vi "Log Setpoints.vi"(8 "error in (no error)":errorcluster, 9 "Time Stamp":timestamp, 10 "Setpoints":T1, 11 "Logger in":refnum<class "Logger.lvclass">) -> (0 "error out":errorcluster, 3 "Logger out":refnum<class "Logger.lvclass">)   [LabVIEW 2015, in "Logger Actor.lvlib" / "Logger.lvclass"]
uses:
  Logger.lvclass
  <vilib>/NI/Tools/Keyed Array/KeyedArray.ctl
  Logger.lvclass/Logger.ctl
  Utilities/Message Strings.llb/Message String Utilities.lvlib
  <vilib>/NI/Tools/Keyed Array/Tools_KeyedArray.lvlib
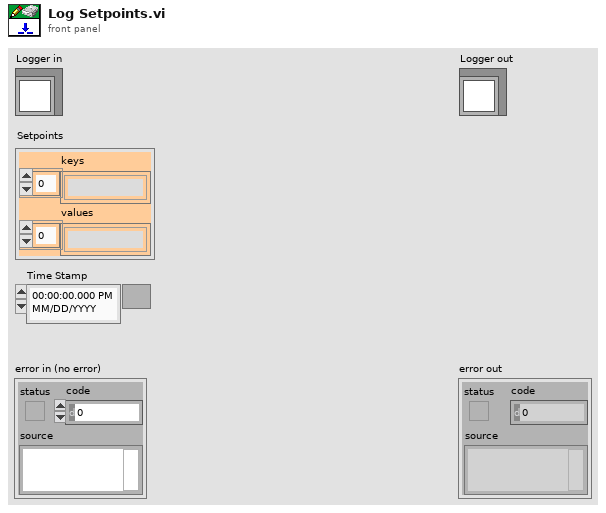
[diagram p1: front panel]
types:
  T1 = typedef "Tools_KeyedArray.lvlib/KeyedArray.ctl" = cluster{"keys":string[], "values":string[]}
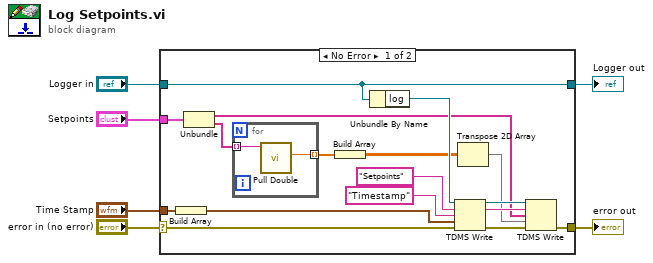
[diagram p0: block diagram]
diagram:
  n1 = case shown="No Error" "error in (no error)" {
    selector: "error in (no error)" -> [w8 w27]
    tunnel: [w12 w27] -> w5
    tunnel: [w23 w26] -> w3
    tunnel: "Logger in" -> [w23 w26]
    tunnel: "Time Stamp" -> [w19 _]
    tunnel: "Setpoints" -> [w15 _]
    frame No Error {
      n2 = Build Array(w19) -> (w18:timestamp[])
      n3 = Unbundle(w15) -> ("keys"=w14:string[], "values"=w11:string[])
      n4 = for {
        tunnel: w11 -> [w25] mode=indexing
        tunnel: [w24] -> w10 mode=indexing
        n5 = call "Pull Double.vi"("String in"=w25) -> ("Double out"=w24:dbl)  [unwired: 8 in, 2 out]
      }
      n6 = Build Array(w10) -> (w9:dbl[][])
      n7 = Unbundle By Name(w23) -> ("log"=w22:refnum<k34>)
      n8 = TDMS Write(0:w22, 5:"Setpoints" ("group name in (Untitled)"), 7:"Timestamp" ("group name in (Untitled)"), 9:w18, 11:w8) -> (4:w17:refnum<k34>, 6:w16:string, 15:w13:errorcluster)  [unwired: 1 in, 1 out]
      n9 = Transpose 2D Array(2D array=w9) -> (transposed array=w7:dbl[][])
      n10 = TDMS Write(0:w17, 5:w16, 7:w14, 9:w7, 11:w13) -> (15:w12:errorcluster)  [unwired: 1 in, 3 out]
    }
    frame Error {
    }
  }
  "error out" <- w5
  "Logger out" <- w3
